vi "Default Path.vi"(8 "error in (no error)":errorcluster, 11 "Generic Client in":refnum<class "Generic Client.lvclass">) -> (0 "error out":errorcluster, 2 "path":path, 3 "Generic Client out":refnum<class "Generic Client.lvclass">)   [LabVIEW 2020, in "NI_SSH.lvlib" / "Generic Client.lvclass"]
uses:
  <vilib>/net/SSH/Client/Generic/Generic Client.lvclass
  <vilib>/Utility/error.llb/Error Cluster From Error Code.vi
  <vilib>/ErrorRing/Error Ring.xnode
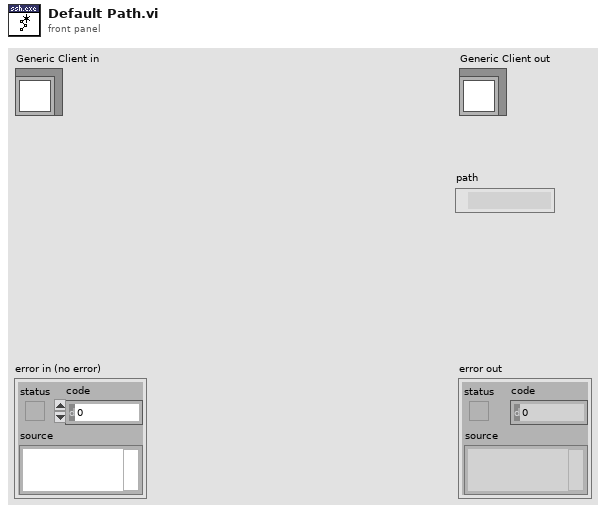
[diagram p1: front panel]
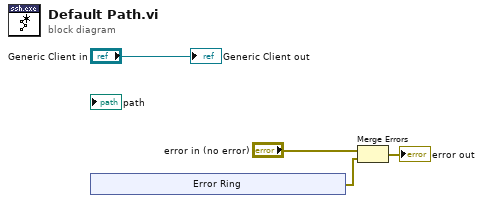
[diagram p0: block diagram]
diagram:
  n1 = xnode ("Error Ring")() -> ("error out"=w2:errorcluster)
  n2 = Merge Errors("error in (no error)", w2) -> (→"error out":errorcluster)
  "Generic Client out" <- "Generic Client in"
